vi "config.vi"(8 "error in (no error)":errorcluster, 10 "Configuration":T1={"Config Dir"=path "/home/ttsai/Documents/stash/ts_tcs_ofc/configData", "Rot Mirror FEA File Name"="rotMat_Bo_to_Chris_FEA_DOF.txt", "Rot Hexapod FEA File Name"="rotMat_hexapod.txt"}, 11 "SubSysAdap in":refnum<class "SubSysAdap.lvclass">) -> (0 "error out":errorcluster, 3 "SubSysAdap out":refnum<class "SubSysAdap.lvclass">)   [LabVIEW 2016, in "OfcFunc.lvlib" / "SubSysAdap.lvclass"]
doc: "Do the configuration of sub-system adaptor (SSA)."
uses:
  SubSysAdap.lvclass
  SubSysAdap.lvclass/SubSysAdap.ctl
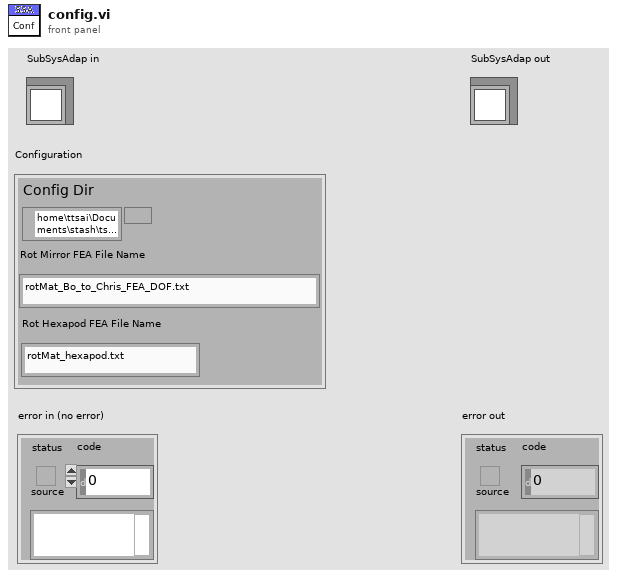
[diagram p1: front panel]
types:
  T1 = cluster{"Config Dir":path, "Rot Mirror FEA File Name":string, "Rot Hexapod FEA File Name":string}
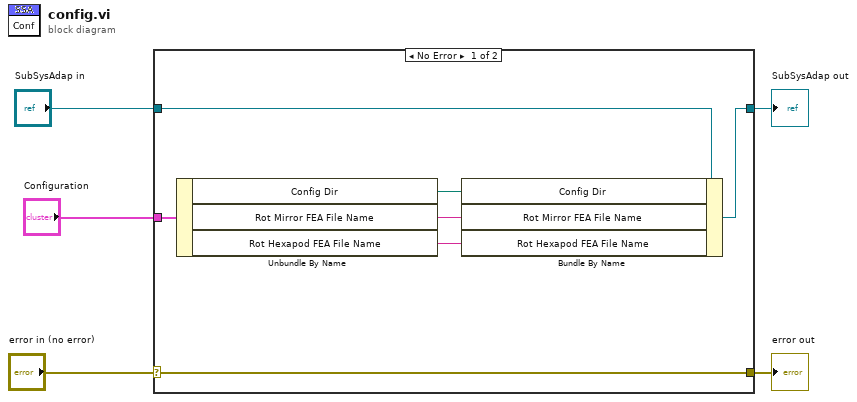
[diagram p0: block diagram]
diagram:
  n1 = case shown="No Error" "error in (no error)" {
    selector: "error in (no error)" -> [w12 w14]
    tunnel: [w12 w14] -> w4
    tunnel: [w9 w13] -> w2
    tunnel: "SubSysAdap in" -> [w10 w13]
    tunnel: "Configuration" -> [w11 _]
    frame No Error {
      n2 = Unbundle By Name(w11) -> ("Config Dir"=w8:path, "Rot Mirror FEA File Name"=w7:string, "Rot Hexapod FEA File Name"=w6:string)
      n3 = Bundle By Name(cluster=w10, "Config Dir"=w8, "Rot Mirror FEA File Name"=w7, "Rot Hexapod FEA File Name"=w6) -> (w9:refnum<class "SubSysAdap.lvclass">)
    }
    frame Error {
    }
  }
  "error out" <- w4
  "SubSysAdap out" <- w2
